vi "Wait For Wavelength Change.vi"(1 "Channel":i32=1) -> ()   [LabVIEW 2020]
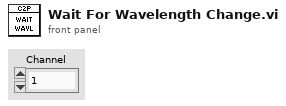
[diagram p1: front panel]
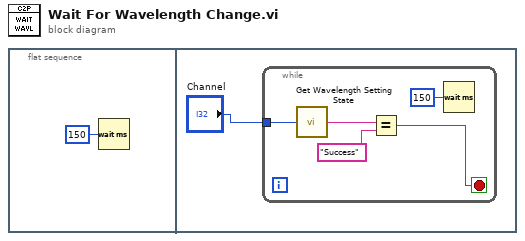
[diagram p0: block diagram]
diagram:
  n1 = flat-sequence {
    frame #0 {
      n2 = Wait (ms)(milliseconds to wait=u32 150) -> ()  [unwired: 1 out]
    }
    frame #1 {
      n3 = while {
        tunnel: "Channel" -> [w7]
        stop <- w4 stop-if-true
        n4 = call "Get Wavelength Setting State.vi"("Channel"=w7) -> ("Wavelength Setting State"=w6:string)
        n5 = Equal?(x=w6, y="Success") -> (x = y?=w4:bool)
        n6 = Wait (ms)(milliseconds to wait=u32 150) -> ()  [unwired: 1 out]
      }
    }
  }
